vi "CastArrayDependenciesToClusterOrClass.vi"(7 "Dependency Type (Class|Cluster)":variant, 8 "error in (no error)":errorcluster, 10 "index (-1: from start)":i32=-1, 11 "[Dependencies]":refnum<class>[](array[class])) -> (0 "error out":errorcluster, 3 "Dependencies output":variant)   [LabVIEW 2021, in "smo.lvlib" / "SMO.lvclass"]
uses:
  SMO.lvclass
  SMO.lvclass/SMO.ctl
  <vilib>/Utility/VariantDataType/VariantType.lvlib
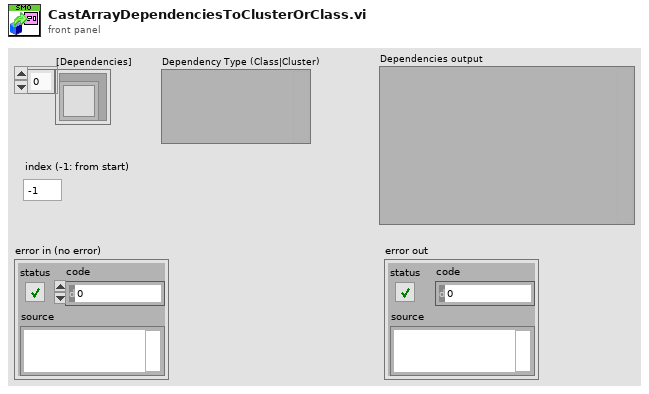
[diagram p1: front panel]
types:
  T1 = typedef "VariantType.lvlib/Type.ctl" = enum8{"Invalid Type", "Void", "I8", "I16", "I32", "I64", "U8", "U16", "U32", "U64", "Single Float", "Double Float", "Extended Float", "Single Complex", "Double Complex", "Extended Complex", "Enum U8", "Enum U16", "Enum U32", "Enum U64", "Single Float With Unit", "Double Float With Unit", "Extended Float With Unit", "Single Complex with Unit", "Double Complex with Unit", "Extended Complex with Unit", "Boolean", "String", "Path", "Picture", "Tag", "Array", "Cluster", "Variant", "LV Variant", "Waveform", "Timestamp", "Digital Waveform", "Digital Data", "ExpressData", "Refnum", "External Data", "VI", "Poly VI", "LabVIEW Class Instance", "Fixed Point"}
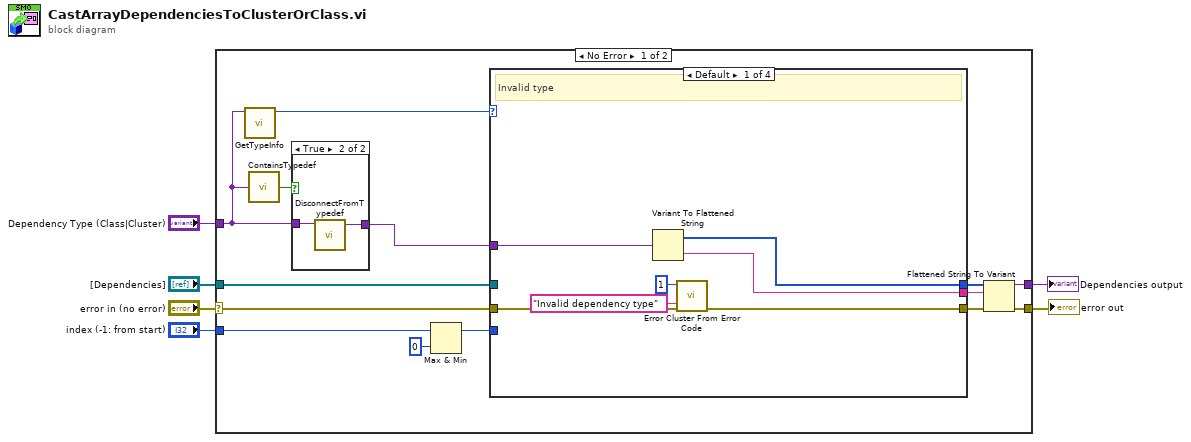
[diagram p0: block diagram]
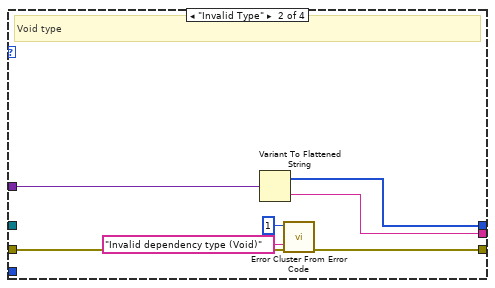
[diagram p3: hidden frame]
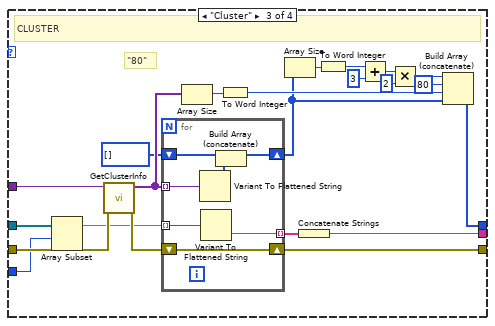
[diagram p4: hidden frame]
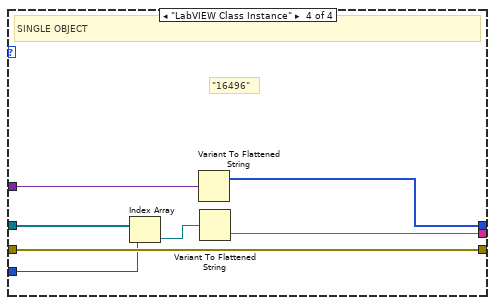
[diagram p5: hidden frame]
diagram:
  n1 = case shown="No Error" "error in (no error)" {
    selector: "error in (no error)" -> [w7 w74]
    tunnel: [w20 w75] -> w6
    tunnel: [w19 w74] -> w5
    tunnel: "[Dependencies]" -> [w17 _]
    tunnel: "index (-1: from start)" -> [w13 _]
    tunnel: "Dependency Type (Class|Cluster)" -> [w9 w75]
    frame No Error {
      n2 = call <vilib>:"GetTypeInfo.vi"("Variant"=w9) -> ("Type Enum"=w8:T1)  [unwired: 6 in, 4 out]
      n3 = call <vilib>:"ContainsTypedef.vi"("lvvar"=w9) -> ("Contains Typedef"=w11:bool)
      n4 = case shown="True" w11 {
        tunnel: w9 -> [w21 w23]
        tunnel: [w21 w22] -> w10
        frame False {
        }
        frame True {
          n5 = call <vilib>:"DisconnectFromTypedef.vi"("lvvar in"=w23) -> ("lvvar out"=w22:variant)  [unwired: 4 in, 1 out]
        }
      }
      n6 = Max & Min(x=w13, y=0) -> (max(x,y)=w12:i32)  [unwired: 1 out]
      n7 = case shown="Default" w8 {
        tunnel: [w26 w33 w59 w72] -> w18
        tunnel: w17 -> [_ _ w40 w69]
        tunnel: w7 -> [w27 w34 w58 w72]
        tunnel: [w28 w35 w51 w70] -> w16
        tunnel: [w29 w36 w43 w71] -> w15
        tunnel: w10 -> [w30 w37 w42 w73]
        tunnel: w12 -> [_ _ w38 w67]
        frame Default {
          # "Invalid type"
          n8 = Variant To Flattened String(Variant=w30) -> (data string=w28:string, 1:w29:i16[])
          n9 = call <vilib>:"Error Cluster From Error Code.vi"("error in (no error)"=w27, "error message (\"\")"="Invalid dependency type" ("error message (\"\")"), "error code (0)"=1) -> ("error out"=w26:errorcluster)  [unwired: 6 in]
        }
        frame "Invalid Type" {
          # "Void type"
          n10 = Variant To Flattened String(Variant=w37) -> (data string=w35:string, 1:w36:i16[])
          n11 = call <vilib>:"Error Cluster From Error Code.vi"("error in (no error)"=w34, "error message (\"\")"="Invalid dependency type (Void)" ("error message (\"\")"), "error code (0)"=1) -> ("error out"=w33:errorcluster)  [unwired: 6 in]
        }
        frame "Cluster" {
          # "\"80\""
          # "CLUSTER"
          n12 = Array Subset(array=w40, index=w38) -> (w39:refnum<class>[])  [unwired: 1 in]
          n13 = call <vilib>:"GetClusterInfo.vi"("error in (no error)"=w58, "Variant"=w42) -> ("error out"=w57:errorcluster, "Cluster Elements"=w56:variant[])  [unwired: 8 in]
          n14 = for {
            tunnel: w39 -> [w66] mode=indexing
            shift-right: [w65] -> w59
            shift-left: w57 -> [w65]
            tunnel: w56 -> [w64] mode=indexing
            shift-right: [w62] -> w44
            shift-left: i16[] [] -> [w63]
            tunnel: [w61] -> w52 mode=indexing
            n15 = Variant To Flattened String(Variant=w64) -> (1:w60:i16[])  [unwired: 1 out]
            n16 = Variant To Flattened String(Variant=w66) -> (data string=w61:string)  [unwired: 1 out]
            n17 = Build Array (concatenate)(w63, w60) -> (w62:i16[])
          }
          n18 = Array Size(array=w56) -> (size(s)=w55:i32)
          n19 = To Word Integer(number=w55) -> (16bit integer=w54:i16)
          n20 = Array Size(array=w44) -> (size(s)=w46:i32)
          n21 = Concatenate Strings(w52) -> (w51:string)
          n22 = To Word Integer(number=w46) -> (16bit integer=w50:i16)
          n23 = Add(x=w50, y=i16 3) -> (x+y=w48:i16)
          n24 = Multiply(x=w48, y=i16 2) -> (x*y=w45:i16)
          n25 = Build Array (concatenate)(w45, i16 80 ("16bit integer"), w54, w44) -> (w43:i16[])
        }
        frame "LabVIEW Class Instance" {
          # "\"16496\""
          # "SINGLE OBJECT"
          n26 = Index Array(array=w69, index=w67) -> (element=w68:refnum<class>)
          n27 = Variant To Flattened String(Variant=w73) -> (1:w71:i16[])  [unwired: 1 out]
          n28 = Variant To Flattened String(Variant=w68) -> (data string=w70:string)  [unwired: 1 out]
        }
      }
      n29 = Flattened String To Variant(4:w18, 6:w16, 7:w15) -> (0:w19:errorcluster, 3:w20:variant)
    }
    frame Error {
    }
  }
  "error out" <- w5
  "Dependencies output" <- w6
